vi "BoxSimArm.vi"() -> ()   [LabVIEW 2023]
uses:
  <vilib>/Rock Robotics/WPI/ThirdParty/JAS_Junk/TrajLib/Enum/DCMOTOR_TYPES_ENUM.ctl
  <vilib>/Rock Robotics/WPI/ThirdParty/JAS_Junk/TrajLib/VI/Util_GetTime_U32.vi
  <vilib>/Rock Robotics/WPI/ThirdParty/JAS_Junk/TrajLib/VI/numCmd_ObtainQueue_OneDbl.vi
  <vilib>/Rock Robotics/WPI/ThirdParty/JAS_Junk/TrajLib/SlewRateLimiter_New.vi
  <vilib>/Rock Robotics/WPI/ThirdParty/JAS_Junk/TrajLib/SlewRateLimiter_Reset.vi
  <vilib>/Rock Robotics/WPI/ThirdParty/JAS_Junk/TrajLib/SlewRateLimiter_Calculate.vi
  <vilib>/Rock Robotics/WPI/ThirdParty/JAS_Junk/TrajLib/SlewRateLimiter_SetRate.vi
  <vilib>/Rock Robotics/WPI/ThirdParty/JAS_Junk/TrajLib/BatterySim_CalculateLoadedBatteryVoltage.vi
  <vilib>/Rock Robotics/WPI/ThirdParty/JAS_Junk/TrajLib/VI/Util_GetTime_U64.vi
  <vilib>/Rock Robotics/WPI/ThirdParty/JAS_Junk/TrajLib/Trajectory_Library.lvlib
panel:
  out "Gravity Comp Output":dbl
  out "Motor Current":dbl
  out "Rev / Lo Lim":bool
  out "Fwd / Hi Lim":bool
  out "Arm Demand Deg":dbl
  out "Battery Voltage":dbl format="%10.1f"
  out "Shooter Control":T1(graph)
  out "Position DEG":dbl format="%13.1f"
  out "AtSetpoint":bool
  in  "Pos Dmd DEG":dbl=90.0 min=-36.0 max=150.0 step=2.5
  out "Motor Dmd (CO)":dbl format="%10.3f"
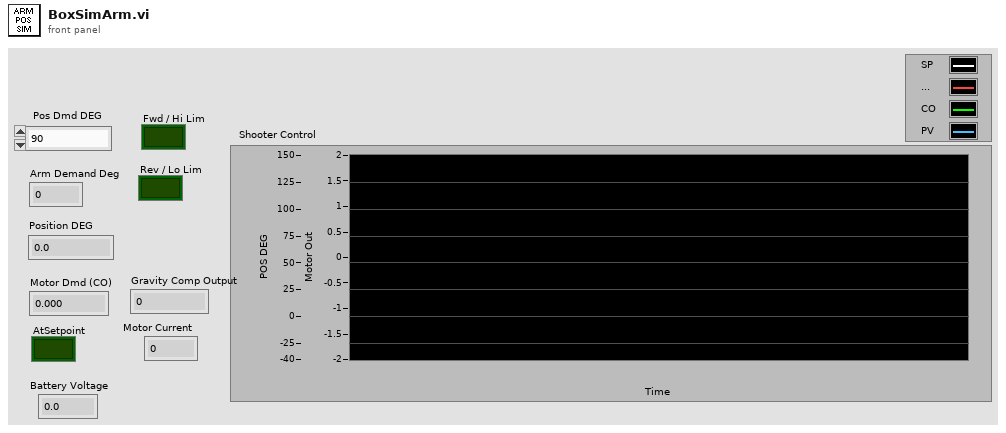
[diagram p1: front panel]
types:
  T1 = cluster{"Setpoint":dbl, "FeedForward":dbl, "CO-ControlOutput":dbl, "Velocity_RPM":dbl}
  T2 = typedef "Trajectory_Library.lvlib/DCMOTOR_TYPES_ENUM.ctl" = enum16{"CIM", "AndyMark 9015", "Andy Mark RS 775 125", "Bag", "BaneBots RS 550", "BaneBots RS 775", "Falcon 500", "Mini CIM", "NEO", "NEO 550", "Romi BuiltIn", "Vex 775 Pro", "Snow Blower AM 2235A", "Bosch Seat AM 3493"}
  T3 = typedef "Trajectory_Library.lvlib/LINEAR_SYSTEM_ID_SINGLE_JOINT_ARM_MODEL.ctl" = cluster{"DCMOTOR_TYPES":T2, "Num Motors":i32, "ArmLength_M":dbl, "massKg":dbl, "Gearing":dbl, "MOI kgm2":dbl, "Estimate MOI":bool}
  T4 = typedef "Trajectory_Library.lvlib/SINGLE_JOINT_ARM_SIM_SIMULATION_PARAMS.ctl" = cluster{"MinAngle_Rad":dbl, "MaxAngle_Rad":dbl, "Measurment StdDev":dbl, "SimulateGravity":bool}
  T5 = cluster{"Pos Dmd DEG":dbl, "Arm Demand Deg":dbl, "Motor Output":dbl, "Degrees":dbl}
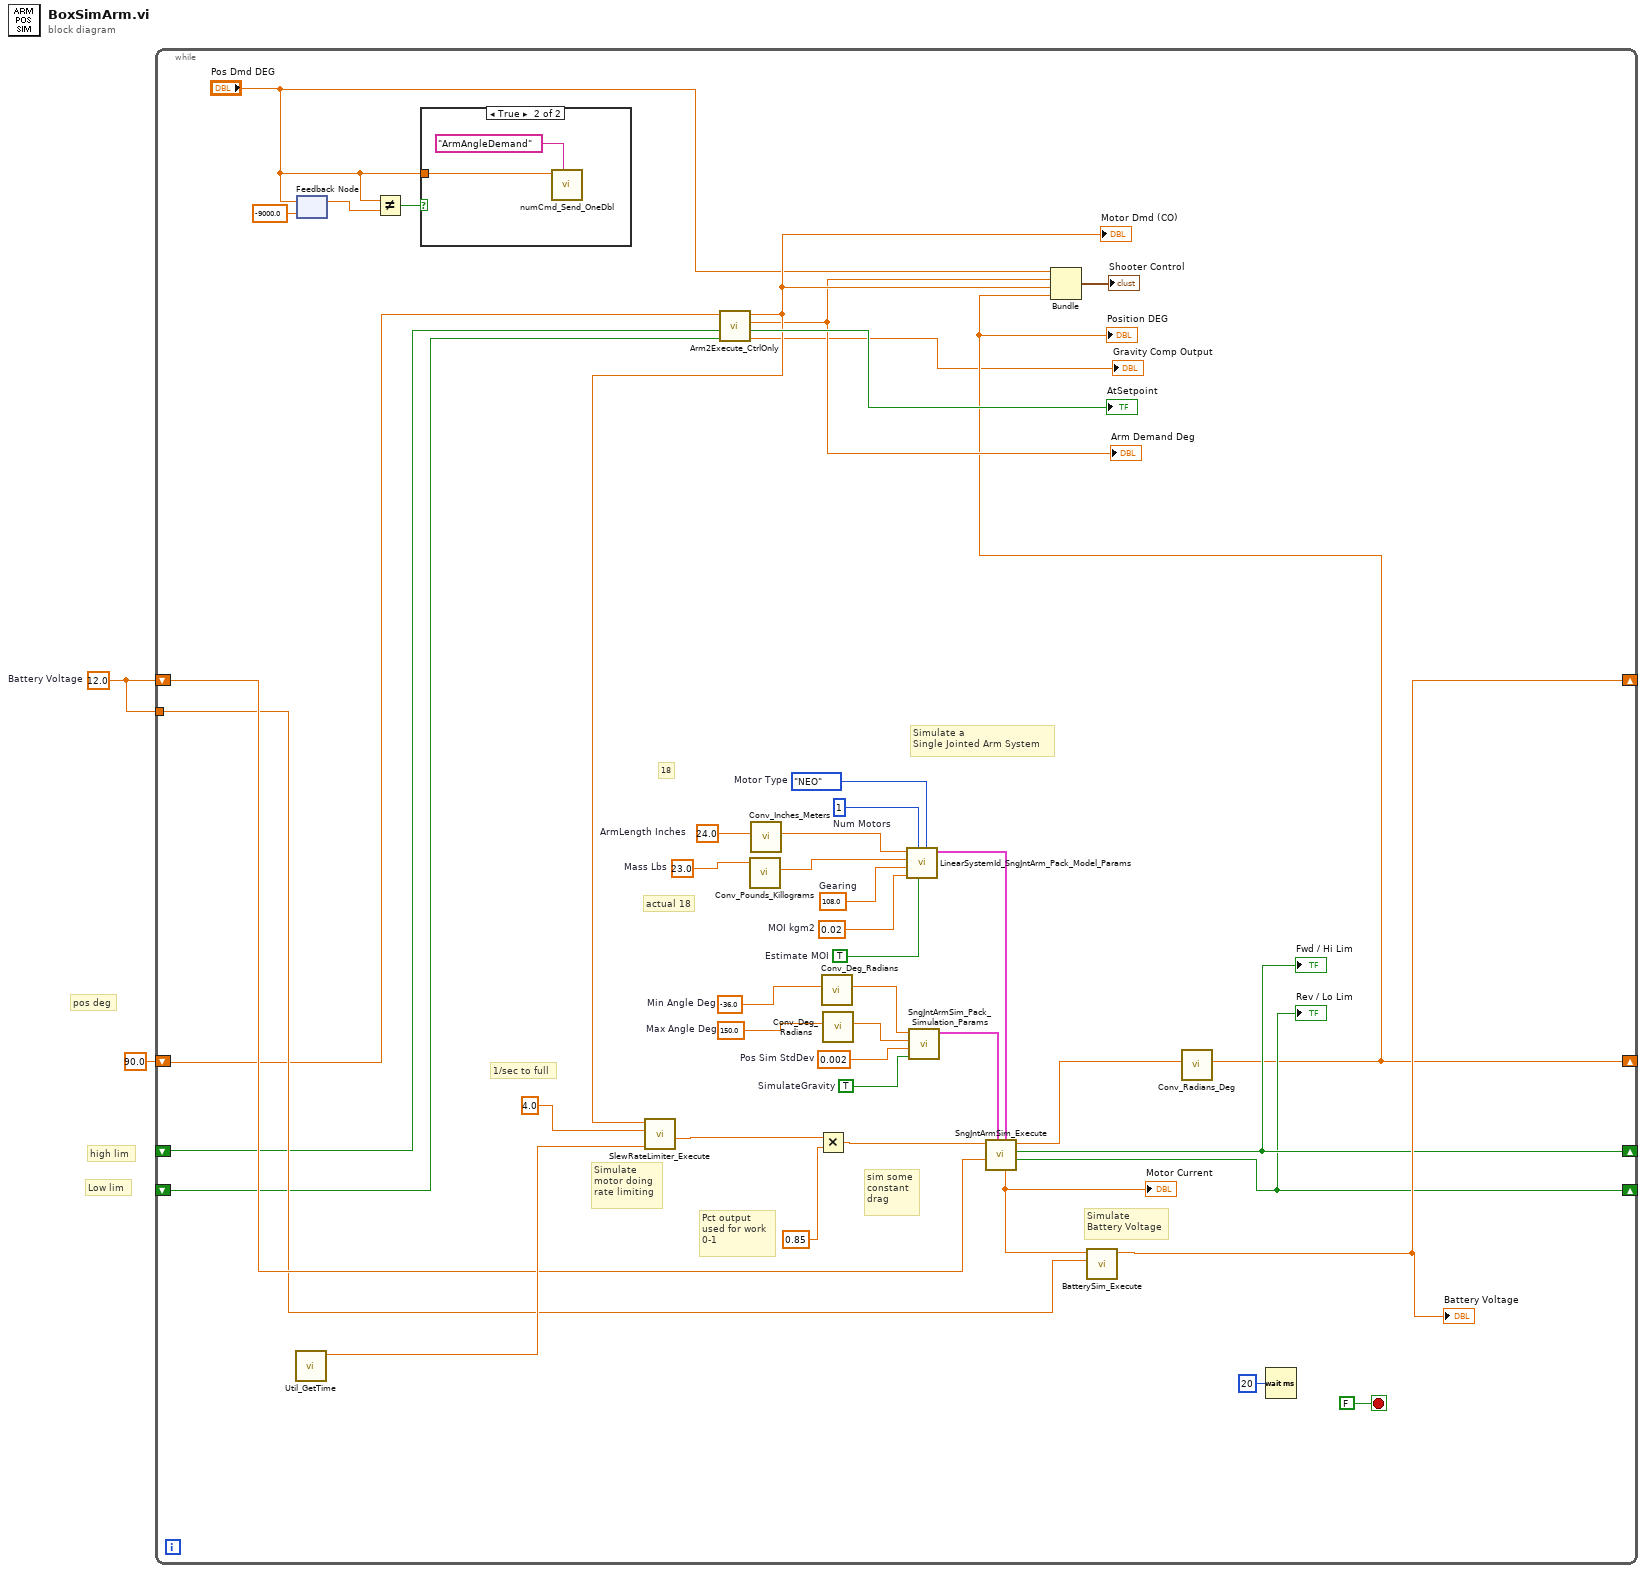
[diagram p0: block diagram]
diagram:
  w2 = 12.0  # Battery Voltage
  # "pos deg"
  # "Low lim"
  # "high lim"
  n1 = while {
    shift-right: [w17] -> _
    shift-left: w2 -> [w29]
    shift-right: [w5] -> _
    shift-left: 90.0 ("Degrees") -> [w13]
    tunnel: w2 -> [w28]
    shift-right: [w7] -> _
    shift-left: _ -> [w12]
    shift-right: [w6] -> _
    shift-left: _ -> [w11]
    stop <- FALSE stop-if-true
    w32 = TRUE  # Estimate MOI
    w33 = 0.02  # MOI kgm2
    w27 = -36.0  # Min Angle Deg
    w26 = 150.0  # Max Angle Deg
    w34 = 0.002  # Pos Sim StdDev
    w35 = TRUE  # SimulateGravity
    w21 = 24.0  # ArmLength Inches
    w37 = 108.0  # Gearing
    w22 = 23.0  # Mass Lbs
    w38 = 1  # Num Motors
    w39 = DCMOTOR_TYPES_ENUM."NEO"  # Motor Type
    # "actual 18"
    # "18"
    # "1/sec to full"
    # "Simulate\nBattery Voltage"
    # "Simulate a\nSingle Jointed Arm System"
    # "Pct output\nused for work\n0-1"
    # "Simulate\nmotor doing\nrate limiting"
    # "sim some\nconstant\ndrag"
    n2 = call <vilib>:"Util_GetTime.vi"() -> ("FPGA_Time_Seconds"=w40:dbl)  [unwired: 9 in, 2 out]
    n3 = feedback-in #1("Pos Dmd DEG") -> ()
    n4 = feedback #1(-9000.0 ("Pos Dmd DEG")) -> (w8:dbl)
    n5 = Not Equal?(x="Pos Dmd DEG", y=w8) -> (x != y?=w10:bool)
    n6 = case shown="True" w10 {
      tunnel: "Pos Dmd DEG" -> [_ w47]
      frame False {
      }
      frame True {
        n7 = call <vilib>:"numCmd_Send_OneDbl.vi"("Command Name"="ArmAngleDemand", "Value"=w47) -> ()  [unwired: 9 in, 1 out]
      }
    }
    n8 = call "Arm2Execute_CtrlOnly.vi"("ReverseLimitSwitch"=w11, "ForwardLimitSwitch"=w12, "SensorPos Deg"=w13) -> ("Gravity Comp Output"=→"Gravity Comp Output":dbl, "OnTarget"=→"AtSetpoint":bool, "Arm Demand Deg"=w14:dbl, "Motor Output"=w15:dbl)  [unwired: 5 in]
    "Motor Dmd (CO)" <- w15
    "Arm Demand Deg" <- w14
    n9 = call <vilib>:"SlewRateLimiter_Execute.vi"("Time"=w40, "PositiveRate"=4.0 ("y"), "Input"=w15) -> ("Output"=w43:dbl)  [unwired: 7 in, 1 out]
    n10 = call <vilib>:"Conv_Pounds_Killograms.vi"("Pounds"=w22) -> ("Killograms"=w23:dbl)  [unwired: 10 in]
    n11 = call <vilib>:"Conv_Inches_Meters.vi"("INCH"=w21) -> ("Meters"=w20:dbl)  [unwired: 10 in]
    n12 = Multiply(x=w43, y=0.85) -> (x*y=w19:dbl)
    n13 = call <vilib>:"Conv_Deg_Radians.vi"("Degress"=w27) -> ("Radians"=w25:dbl)  [unwired: 10 in]
    n14 = call <vilib>:"Conv_Deg_Radians.vi"("Degress"=w26) -> ("Radians"=w24:dbl)  [unwired: 10 in]
    n15 = call <vilib>:"LinearSystemId_SngJntArm_Pack_Model_Params.vi"("DCMOTOR_TYPES"=w39, "Estimate MOI"=w32, "Num Motors"=w38, "MOI kgm2"=w33, "Gearing"=w37, "massKg"=w23, "ArmLength_M"=w20) -> ("SngJntArmSim_Model _Params"=w31:T3)  [unwired: 4 in]
    n16 = call <vilib>:"SngJntArmSim_Pack_Simulation_Params.vi"("SimulateGravity"=w35, "Pos Sim StdDev Rad"=w34, "MaxAngle_Rad"=w24, "MinAngle_Rad"=w25) -> ("SngJntArmSim_Simulation _Params"=w30:T4)  [unwired: 7 in]
    n17 = call <vilib>:"SngJntArmSim_Execute.vi"("SngJntArmSim_Model _Params"=w31, "SngJntArmSim_Simulation _Params"=w30, "Battery Volts"=w29, "Motor Dmd"=w19) -> ("AtLowLimit"=w6:bool, "At HIgh LImit"=w7:bool, "ArmAngle_Rad"=w18:dbl, "Motor Current"=w36:dbl)  [unwired: 2 in, 2 out]
    "Fwd / Hi Lim" <- w7
    "Rev / Lo Lim" <- w6
    "Motor Current" <- w36
    n18 = call <vilib>:"BatterySim_Execute.vi"("Nominal Battery Voltage"=w28, "Current"=w36) -> ("Voltage"=w17:dbl)  [unwired: 9 in]
    "Battery Voltage" <- w17
    n19 = call <vilib>:"Conv_Radians_Deg.vi"("Radians"=w18) -> ("Degrees"=w5:dbl)  [unwired: 10 in]
    "Position DEG" <- w5
    n20 = Bundle("Pos Dmd DEG"="Pos Dmd DEG", "Arm Demand Deg"=w14, "Motor Output"=w15, "Degrees"=w5) -> (→"Shooter Control":T5)  [unwired: 1 in]
    n21 = Wait (ms)(milliseconds to wait=u32 20) -> ()  [unwired: 1 out]
  }
